vi "COM.vi"(11 "Array":string[](array[string])=["COM1", "H", "L", "", "", "", "", ""]) -> (3 "Array 3":string[](array[string])=["COM1", "H", "L", "", "", "", "", ""])   [LabVIEW 2013]
panel:
  in  "Test Item":string="write snSDFSF"
  in  "Lolimits":string="000"
  in  "Uplimits":string="55"
  in  "Sent data":string="SDFDAFA"
  in  "Baud rate":string(combo)="9600"
  in  "Data bits":string(combo)="8"
  in  "VISA  name":refnum<visa-resource-name>="COM1"
  in  "Parity":string(combo)="None"
  in  "Stop Button":bool
  in  "OK Button":bool
  out "element 5":string
  out "element 4":string
  out "element 3":string="L"
  out "element 2":string="H"
  out "element":string="COM1"
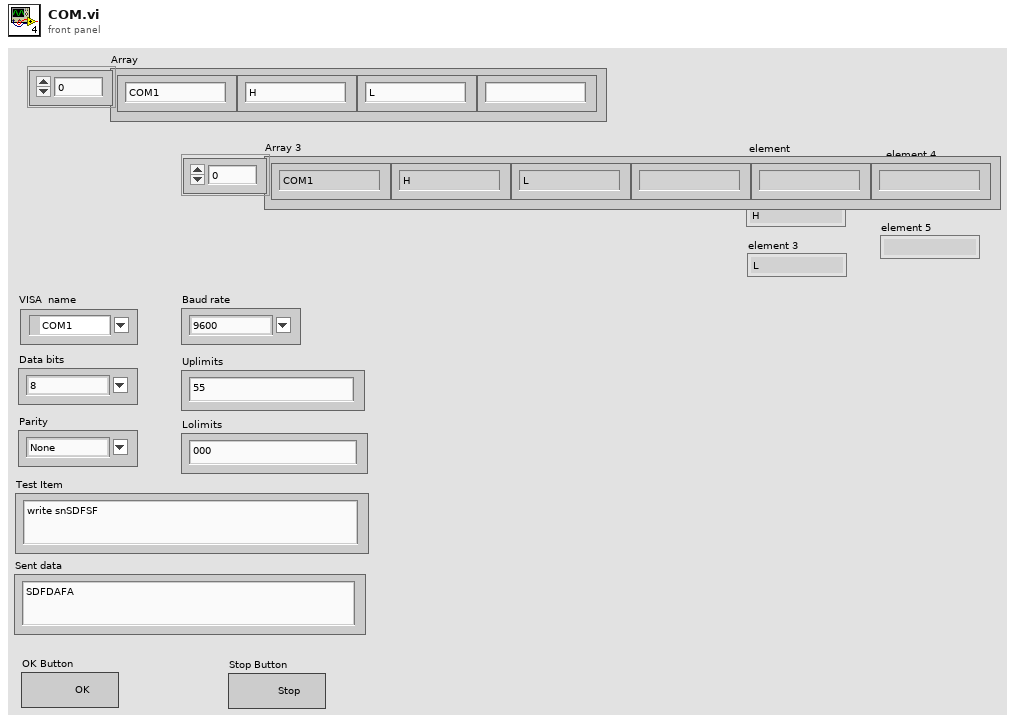
[diagram p1: front panel]
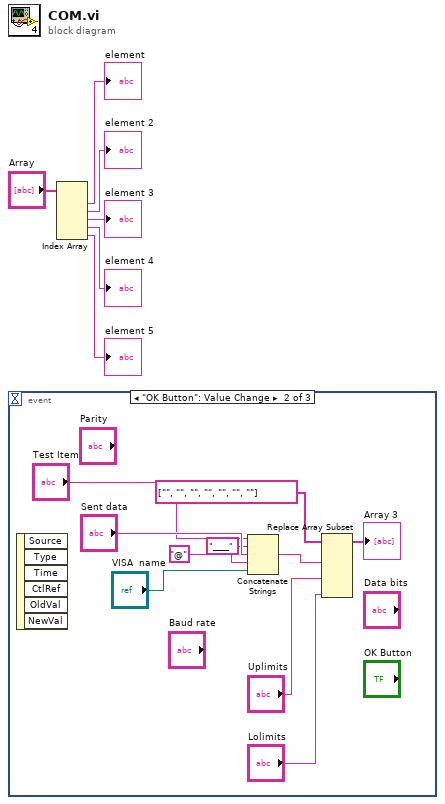
[diagram p0: block diagram]
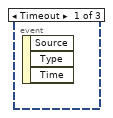
[diagram p2: hidden frame]
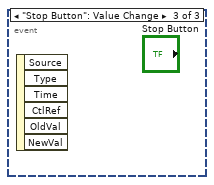
[diagram p3: hidden frame]
diagram:
  n1 = event shown="[1] \"OK Button\": Value Change" {
    selector: _ -> [_ _ _]
    dyn-events: _ -> [_ _ _]
    timeout: _ -> [_ _ _]
    event Timeout {
      n2 = event-data() -> ()  [unwired: 1 in, 3 out]
    }
    event "OK Button": Value Change {
      n3 = event-data() -> ()  [unwired: 1 in, 6 out]
      n4 = Concatenate Strings("Test Item", "____" ("string"), "Sent data", "@" ("string"), "VISA  name") -> (w16:string)
      n5 = Replace Array Subset(array=string[] ["", "", "", "", "", "", ""], new element #1=w16, new element #2="Uplimits", new element #3="Lolimits") -> (→"Array 3":string[])  [unwired: 3 in]
    }
    event "Stop Button": Value Change {
      n6 = event-data() -> ()  [unwired: 1 in, 6 out]
    }
  }
  n7 = Index Array(array="Array") -> (element #1=→"element":string, element #2=→"element 2":string, element #3=→"element 3":string, element #4=→"element 4":string, element #5=→"element 5":string)  [unwired: 5 in]
